vi "Bezier1.vi"(2 "d":dbl=3.0, 4 "y":dbl=3.0, 5 "x":dbl=3.0, 6 "Y":dbl[](array[numeric]), 7 "X":dbl[](array[numeric])) -> (0 "查询的y":dbl[](array[numeric]) format="%.3g", 1 "待查找值":dbl[](array[numeric]))   [LabVIEW 2012]
panel:
  out "XY Graph":cluster{"x":dbl[], "y":dbl[]}[](graph) caption="XY图"
  # "查询范围："
  # "~"
  # "间隔："
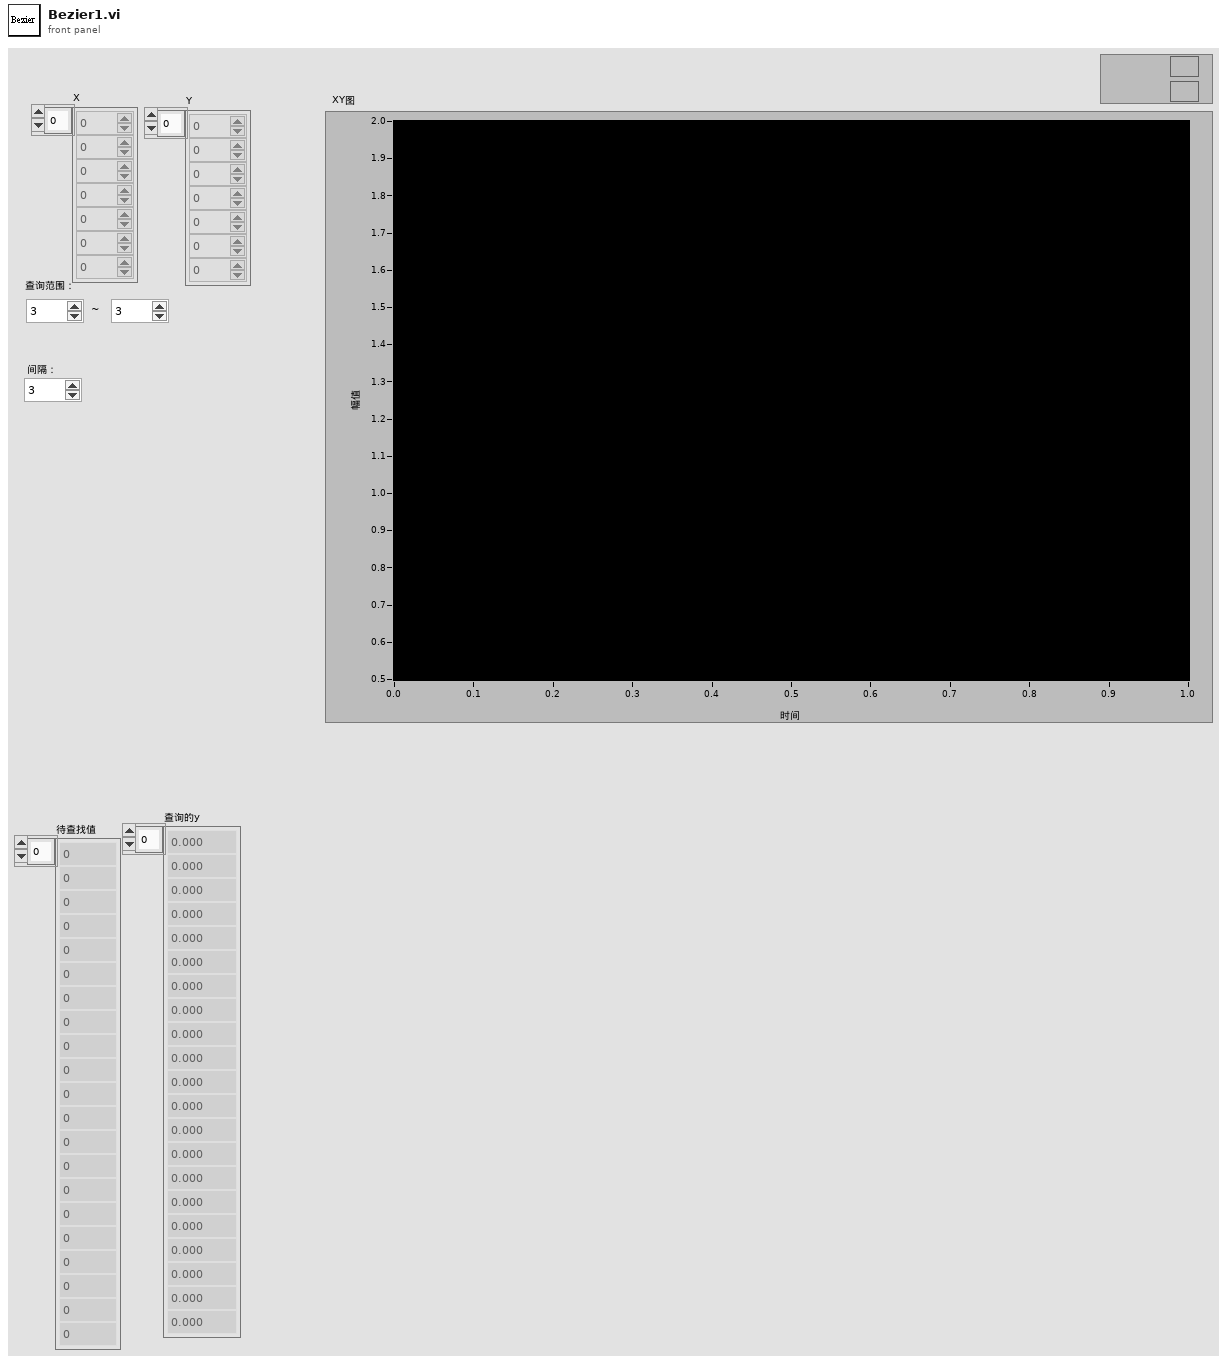
[diagram p1: front panel]
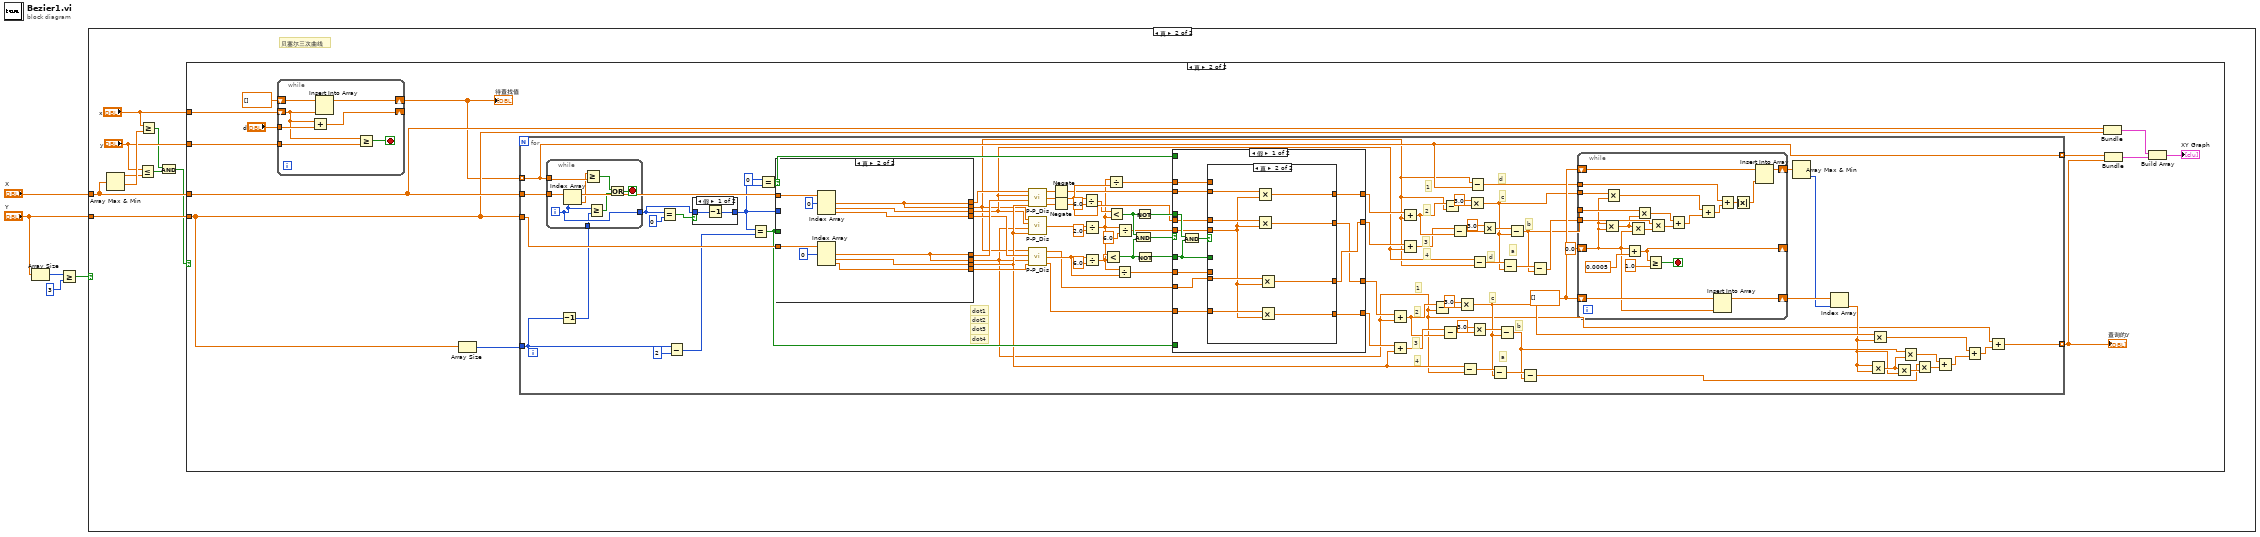
[diagram p0: block diagram]
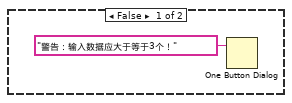
[diagram p2: hidden frame]
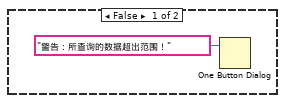
[diagram p3: hidden frame]
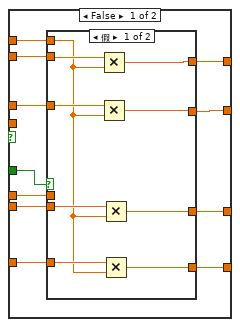
[diagram p5: hidden frame]
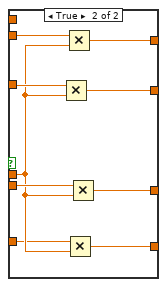
[diagram p6: hidden frame]
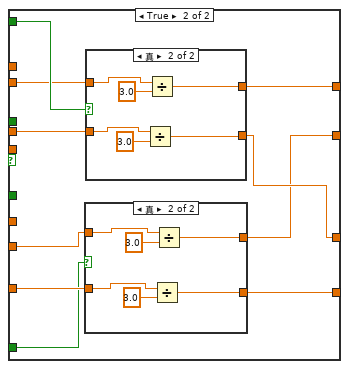
[diagram p7: hidden frame]
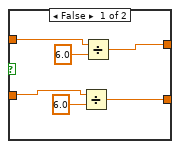
[diagram p8: hidden frame]
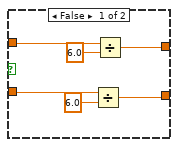
[diagram p9: hidden frame]
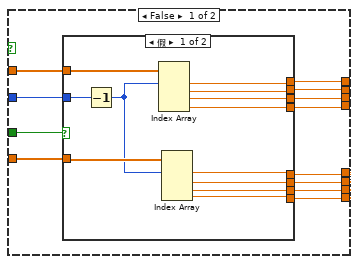
[diagram p10: hidden frame]
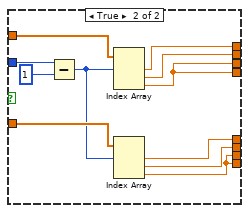
[diagram p11: hidden frame]
diagram:
  n1 = Array Size(array="Y") -> (size(s)=w3:i32)
  n2 = Greater Or Equal?(x=w3, y=3) -> (x >= y?=w1:bool)
  n3 = case shown="真" w1 {
    tunnel: "X" -> [_ w14]
    tunnel: "Y" -> [_ w15]
    frame False {
      n4 = One Button Dialog(message="警告：输入数据应大于等于3个！" ("消息")) -> ()  [unwired: 1 in, 1 out]
    }
    frame True {
      # "贝塞尔三次曲线"
      n5 = Array Max & Min(array=w14) -> (max value=w10:dbl, min value=w12:dbl)  [unwired: 2 out]
      n6 = Less Or Equal?(x="y", y=w10) -> (x <= y?=w8:bool)
      n7 = Greater Or Equal?(x="x", y=w12) -> (x >= y?=w9:bool)
      n8 = And(x=w9, y=w8) -> (x .and. y?=w7:bool)
      n9 = case shown="真" w7 {
        tunnel: "x" -> [_ w28]
        tunnel: "y" -> [_ w27]
        tunnel: w14 -> [_ w24]
        tunnel: w15 -> [_ w23]
        frame False {
          n10 = One Button Dialog(message="警告：所查询的数据超出范围！" ("消息")) -> ()  [unwired: 1 in, 1 out]
        }
        frame True {
          n11 = while {
            tunnel: w27 -> [w285]
            tunnel: "d" -> [w289]
            shift-right: [w286] -> _
            shift-left: w28 -> [w283]
            shift-right: [w288] -> w17
            shift-left: dbl[] [] -> [w287]
            stop <- w284 stop-if-true
            n12 = Add(x=w283, y=w289) -> (x+y=w286:dbl)
            n13 = Insert Into Array(array=w287, new element=w283) -> (w288:dbl[])  [unwired: 1 in]
            n14 = Greater Or Equal?(x=w283, y=w285) -> (x >= y?=w284:bool)
          }
          "待查找值" <- w17
          n15 = Array Size(array=w23) -> (size(s)=w29:i32)
          n16 = for {
            tunnel: w24 -> [w95]
            tunnel: w23 -> [w94]
            tunnel: w29 -> [w36]
            tunnel: w17 -> [w67] mode=indexing
            tunnel: [w67] -> w22 mode=indexing
            tunnel: [w47] -> w19 mode=indexing
            w64 = dbl[] [] ("数组")
            # "1"
            # "2"
            # "3"
            # "4"
            # "d"
            # "c"
            # "b"
            # "a"
            # "1"
            # "2"
            # "3"
            # "4"
            # "dot4"
            # "dot2"
            # "dot3"
            # "dot1"
            # "d"
            # "c"
            # "b"
            # "a"
            n17 = Decrement(x=w36) -> (x-1=w35:i32)
            n18 = while {
              tunnel: w67 -> [w127]
              tunnel: w95 -> [w129]
              tunnel: [w125] -> w31
              tunnel: w35 -> [w124]
              i -> [w125]
              stop <- w128 stop-if-true
              n19 = Index Array(array=w129, index=w125) -> (element=w126:dbl)
              n20 = Greater Or Equal?(x=w126, y=w127) -> (x >= y?=w122:bool)
              n21 = Greater Or Equal?(x=w125, y=w124) -> (x >= y?=w123:bool)
              n22 = Or(x=w122, y=w123) -> (x .or. y?=w128:bool)
            }
            n23 = Equal?(x=w31, y=0 ("x")) -> (x = y?=w32:bool)
            n24 = Subtract(x=w36, y=2) -> (x-y=w40:i32)
            n25 = case shown="假" w32 {
              tunnel: w31 -> [w120 w121]
              tunnel: [w119 w121] -> w30
              frame False {
                n26 = Decrement(x=w120) -> (x-1=w119:i32)
              }
              frame True {
              }
            }
            n27 = Equal?(x=w30, y=w40) -> (x = y?=w83:bool)
            n28 = Equal?(x=0, y=w30) -> (x = y?=w111:bool)
            n29 = case shown="真" w111 {
              tunnel: [w246 w281] -> w97
              tunnel: [w244 w281] -> w44
              tunnel: [w243 w280] -> w66
              tunnel: [w242 w275] -> w98
              tunnel: [w248 w278] -> w117
              tunnel: [w247 w278] -> w34
              tunnel: [w245 w276] -> w81
              tunnel: [w249 w277] -> w113
              tunnel: w95 -> [w241 w282]
              tunnel: w94 -> [w240 w279]
              tunnel: w30 -> [w238 _]
              tunnel: w83 -> [w239 _]
              frame False {
                n30 = case shown="假" w239 {
                  tunnel: [w252 w267] -> w249
                  tunnel: [w255 w265] -> w248
                  tunnel: [w254 w264] -> w247
                  tunnel: [w260 w269] -> w246
                  tunnel: [w259 w268] -> w244
                  tunnel: [w253 w267] -> w245
                  tunnel: [w258 w270] -> w243
                  tunnel: [w257 w270] -> w242
                  tunnel: w238 -> [w251 w262]
                  tunnel: w241 -> [w261 w271]
                  tunnel: w240 -> [w256 w266]
                  frame False {
                    n31 = Decrement(x=w251) -> (x-1=w250:i32)
                    n32 = Index Array(array=w261, index #1=w250) -> (element #1=w260:dbl, element #2=w259:dbl, element #3=w258:dbl, element #4=w257:dbl)  [unwired: 3 in]
                    n33 = Index Array(array=w256, index #1=w250) -> (element #1=w255:dbl, element #2=w254:dbl, element #3=w253:dbl, element #4=w252:dbl)  [unwired: 3 in]
                  }
                  frame True {
                    n34 = Subtract(x=w262, y=1) -> (x-y=w263:i32)
                    n35 = Index Array(array=w271, index #1=w263) -> (element #1=w269:dbl, element #2=w268:dbl, element #3=w270:dbl)  [unwired: 2 in]
                    n36 = Index Array(array=w266, index #1=w263) -> (element #1=w265:dbl, element #2=w264:dbl, element #3=w267:dbl)  [unwired: 2 in]
                  }
                }
              }
              frame True {
                n37 = Index Array(array=w279, index #1=0 ("索引")) -> (element #1=w278:dbl, element #2=w276:dbl, element #3=w277:dbl)  [unwired: 2 in]
                n38 = Index Array(array=w282, index #1=0 ("索引")) -> (element #1=w281:dbl, element #2=w280:dbl, element #3=w275:dbl)  [unwired: 2 in]
              }
            }
            n39 = call "P-P_Dis.vi"("y2"=w81, "y1"=w117, "x2"=w66, "x1"=w97) -> ("y"=w85:dbl, "Dis"=w100:dbl, "x"=w87:dbl)
            n40 = call "P-P_Dis.vi"("y2"=w81, "y1"=w34, "x2"=w66, "x1"=w44) -> ("Dis"=w114:dbl)  [unwired: 2 out]
            n41 = call "P-P_Dis.vi"("y2"=w113, "y1"=w34, "x2"=w98, "x1"=w44) -> ("y"=w37:dbl, "Dis"=w102:dbl, "x"=w38:dbl)
            n42 = Negate(x=w87) -> (-x=w86:dbl)
            n43 = Negate(x=w85) -> (-x=w84:dbl)
            n44 = Divide(x=w100, y=6.0) -> (x/y=w43:dbl)
            n45 = Divide(x=w114, y=2.0) -> (x/y=w42:dbl)
            n46 = Divide(x=w102, y=6.0) -> (x/y=w109:dbl)
            n47 = Less?(x=w109, y=w42) -> (x < y?=w110:bool)
            n48 = Divide(x=w42, y=w100) -> (x/y=w99:dbl)
            n49 = Less?(x=w43, y=w42) -> (x < y?=w106:bool)
            n50 = Divide(x=w42, y=w102) -> (x/y=w101:dbl)
            n51 = Divide(x=w42, y=6.0) -> (x/y=w103:dbl)
            n52 = And(x=w106, y=w110) -> (x .and. y?=w107:bool)
            n53 = Not(x=w106) -> (.not. x?=w105:bool)
            n54 = Not(x=w110) -> (.not. x?=w108:bool)
            n55 = case shown="假" w107 {
              tunnel: w111 -> [_ w213]
              tunnel: w38 -> [w159 w207]
              tunnel: w37 -> [w158 w212]
              tunnel: w86 -> [w162 w211]
              tunnel: w84 -> [w160 w206]
              tunnel: w108 -> [w156 _]
              tunnel: w105 -> [w165 _]
              tunnel: w103 -> [w163 _]
              tunnel: [w161 w210] -> w68
              tunnel: [w153 w204] -> w69
              tunnel: [w152 w205] -> w39
              tunnel: [w157 w209] -> w96
              tunnel: w101 -> [w155 _]
              tunnel: w99 -> [w154 _]
              tunnel: w83 -> [_ w208]
              frame False {
                n56 = And(x=w165, y=w156) -> (x .and. y?=w164:bool)
                n57 = case shown="真" w164 {
                  tunnel: w163 -> [_ w196]
                  tunnel: w162 -> [w172 w203]
                  tunnel: [w170 w202] -> w161
                  tunnel: w160 -> [w171 w201]
                  tunnel: [w169 w200] -> w152
                  tunnel: w159 -> [w175 w199]
                  tunnel: [w168 w198] -> w153
                  tunnel: w158 -> [w174 w197]
                  tunnel: [w167 w195] -> w157
                  tunnel: w156 -> [w176 _]
                  tunnel: w155 -> [w173 _]
                  tunnel: w154 -> [w166 _]
                  frame False {
                    n58 = case shown="假" w176 {
                      tunnel: w175 -> [w181 w190]
                      tunnel: w174 -> [w179 w186]
                      tunnel: w173 -> [_ w187]
                      tunnel: w172 -> [w185 w194]
                      tunnel: w171 -> [w183 w192]
                      tunnel: [w184 w193] -> w170
                      tunnel: [w182 w191] -> w169
                      tunnel: [w180 w189] -> w168
                      tunnel: [w178 w188] -> w167
                      tunnel: w166 -> [w177 _]
                      frame False {
                        n59 = Multiply(x=w185, y=w177) -> (x*y=w184:dbl)
                        n60 = Multiply(x=w183, y=w177) -> (x*y=w182:dbl)
                        n61 = Multiply(x=w181, y=w177) -> (x*y=w180:dbl)
                        n62 = Multiply(x=w179, y=w177) -> (x*y=w178:dbl)
                      }
                      frame True {
                        n63 = Multiply(x=w192, y=w187) -> (x*y=w191:dbl)
                        n64 = Multiply(x=w194, y=w187) -> (x*y=w193:dbl)
                        n65 = Multiply(x=w186, y=w187) -> (x*y=w188:dbl)
                        n66 = Multiply(x=w190, y=w187) -> (x*y=w189:dbl)
                      }
                    }
                  }
                  frame True {
                    n67 = Multiply(x=w203, y=w196) -> (x*y=w202:dbl)
                    n68 = Multiply(x=w201, y=w196) -> (x*y=w200:dbl)
                    n69 = Multiply(x=w199, y=w196) -> (x*y=w198:dbl)
                    n70 = Multiply(x=w197, y=w196) -> (x*y=w195:dbl)
                  }
                }
              }
              frame True {
                n71 = case shown="真" w208 {
                  tunnel: w207 -> [w217 w223]
                  tunnel: w212 -> [w214 w221]
                  tunnel: [w216 w222] -> w204
                  tunnel: [w215 w220] -> w209
                  frame False {
                    n72 = Divide(x=w214, y=6.0) -> (x/y=w215:dbl)
                    n73 = Divide(x=w217, y=6.0) -> (x/y=w216:dbl)
                  }
                  frame True {
                    n74 = Divide(x=w221, y=3.0) -> (x/y=w220:dbl)
                    n75 = Divide(x=w223, y=3.0) -> (x/y=w222:dbl)
                  }
                }
                n76 = case shown="真" w213 {
                  tunnel: w211 -> [w229 w234]
                  tunnel: w206 -> [w227 w237]
                  tunnel: [w228 w233] -> w210
                  tunnel: [w226 w232] -> w205
                  frame False {
                    n77 = Divide(x=w227, y=6.0) -> (x/y=w226:dbl)
                    n78 = Divide(x=w229, y=6.0) -> (x/y=w228:dbl)
                  }
                  frame True {
                    n79 = Divide(x=w237, y=3.0) -> (x/y=w232:dbl)
                    n80 = Divide(x=w234, y=3.0) -> (x/y=w233:dbl)
                  }
                }
              }
            }
            n81 = Add(x=w39, y=w34) -> (x+y=w80:dbl)
            n82 = Add(x=w96, y=w81) -> (x+y=w82:dbl)
            n83 = Add(x=w68, y=w44) -> (x+y=w77:dbl)
            n84 = Add(x=w69, y=w66) -> (x+y=w76:dbl)
            n85 = Subtract(x=w80, y=w34) -> (x-y=w91:dbl)
            n86 = Subtract(x=w82, y=w80) -> (x-y=w88:dbl)
            n87 = Subtract(x=w77, y=w44) -> (x-y=w72:dbl)
            n88 = Subtract(x=w76, y=w77) -> (x-y=w75:dbl)
            n89 = Multiply(x=3.0, y=w91) -> (x*y=w48:dbl)
            n90 = Subtract(x=w81, y=w34) -> (x-y=w89:dbl)
            n91 = Multiply(x=3.0, y=w72) -> (x*y=w61:dbl)
            n92 = Subtract(x=w44, y=w67) -> (x-y=w60:dbl)
            n93 = Subtract(x=w66, y=w44) -> (x-y=w74:dbl)
            n94 = Multiply(x=3.0, y=w88) -> (x*y=w90:dbl)
            n95 = Multiply(x=3.0, y=w75) -> (x*y=w73:dbl)
            n96 = Subtract(x=w89, y=w48) -> (x-y=w79:dbl)
            n97 = Subtract(x=w90, y=w48) -> (x-y=w49:dbl)
            n98 = Subtract(x=w74, y=w61) -> (x-y=w78:dbl)
            n99 = Subtract(x=w73, y=w61) -> (x-y=w62:dbl)
            n100 = Subtract(x=w79, y=w49) -> (x-y=w46:dbl)
            n101 = Subtract(x=w78, y=w62) -> (x-y=w63:dbl)
            n102 = while {
              shift-right: [w151] -> w58
              shift-left: w64 -> [w150]
              shift-right: [w132] -> _
              shift-left: 0.0 ("x") -> [w138]
              shift-right: [w148] -> w59
              shift-left: w64 -> [w147]
              tunnel: w63 -> [w145]
              tunnel: w62 -> [w142]
              tunnel: w61 -> [w139]
              tunnel: w60 -> [w135]
              stop <- w130 stop-if-true
              n103 = Multiply(x=w138, y=w138) -> (x*y=w143:dbl)
              n104 = Multiply(x=w139, y=w138) -> (x*y=w137:dbl)
              n105 = Add(x=w138, y=0.0005) -> (x+y=w132:dbl)
              n106 = Multiply(x=w143, y=w138) -> (x*y=w146:dbl)
              n107 = Multiply(x=w142, y=w143) -> (x*y=w141:dbl)
              n108 = Greater Or Equal?(x=w132, y=1.0) -> (x >= y?=w130:bool)
              n109 = Multiply(x=w145, y=w146) -> (x*y=w144:dbl)
              n110 = Add(x=w141, y=w144) -> (x+y=w140:dbl)
              n111 = Add(x=w137, y=w140) -> (x+y=w136:dbl)
              n112 = Insert Into Array(array=w150, new element=w138) -> (w151:dbl[])  [unwired: 1 in]
              n113 = Add(x=w135, y=w136) -> (x+y=w134:dbl)
              n114 = Absolute Value(x=w134) -> (abs(x)=w133:dbl)
              n115 = Insert Into Array(array=w147, new element=w133) -> (w148:dbl[])  [unwired: 1 in]
            }
            n116 = Array Max & Min(array=w59) -> (min index (indices)=w57:i32)  [unwired: 3 out]
            n117 = Index Array(array=w58, index=w57) -> (element=w45:dbl)
            n118 = Multiply(x=w45, y=w45) -> (x*y=w52:dbl)
            n119 = Multiply(x=w48, y=w45) -> (x*y=w55:dbl)
            n120 = Multiply(x=w52, y=w45) -> (x*y=w50:dbl)
            n121 = Multiply(x=w49, y=w52) -> (x*y=w53:dbl)
            n122 = Multiply(x=w46, y=w50) -> (x*y=w51:dbl)
            n123 = Add(x=w53, y=w51) -> (x+y=w54:dbl)
            n124 = Add(x=w55, y=w54) -> (x+y=w56:dbl)
            n125 = Add(x=w34, y=w56) -> (x+y=w47:dbl)
          }
          "查询的y" <- w19
          n126 = Bundle("X"=w24, "Y"=w23) -> (w21:cluster{"X":dbl[], "Y":dbl[]})  [unwired: 1 in]
          n127 = Bundle(w22, w19) -> (w20:cluster{dbl[], dbl[]})  [unwired: 1 in]
          n128 = Build Array(w21, w20) -> (→"XY Graph":cluster{"X":dbl[], "Y":dbl[]}[])
        }
      }
    }
  }
